vi "Procesado_Matriz.vi"(8 "error in (no error)":errorcluster, 11 "data in":string) -> (0 "error out":errorcluster, 1 "element":u32, 2 "subarray 2":u16[](array[numeric]), 3 "subarray":u16[](array[numeric]))   [LabVIEW 2024]
panel:
  in  "data includes array or string size? (T)":bool=TRUE
  out "*(type *) &x 2":u16[](array[numeric])
  out "*(type *) &x":u8[](array[numeric])
  out "length":i32
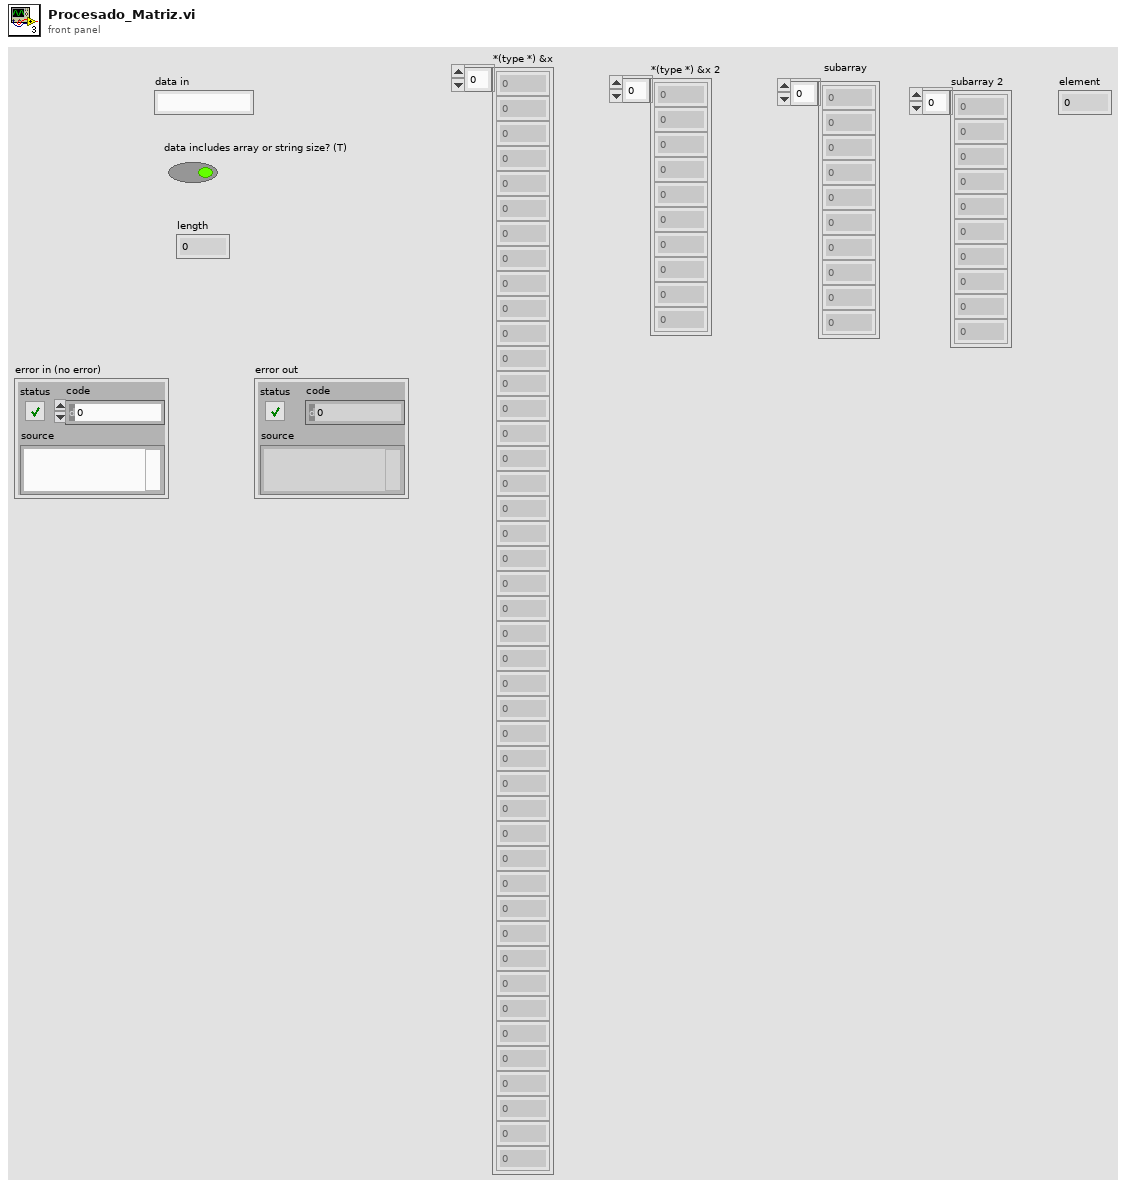
[diagram p1: front panel]
types:
  T1 = enum16{"big-endian, network order", "native, host order", "little-endian"}
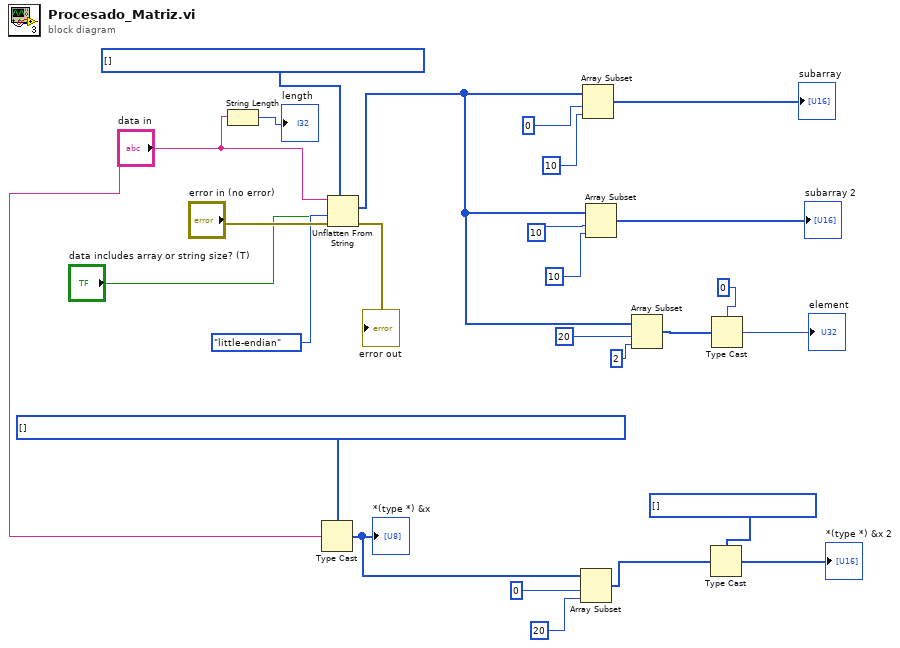
[diagram p0: block diagram]
diagram:
  n1 = String Length(string="data in") -> (length=→"length":i32)
  n2 = Type Cast(type=u8[] [], x="data in") -> (*(type *) &x=w7:u8[])
  "*(type *) &x" <- w7
  n3 = Unflatten From String(type=u16[] [], binary string="data in", data includes array or string size? (T)="data includes array or string size? (T)", byte order (0:big-endian, network order)=T1."little-endian", error in (no error)="error in (no error)") -> (value=w6:u16[], error out=→"error out":errorcluster)  [unwired: 1 out]
  n4 = Array Subset(array=w7, index=0, length=20) -> (w11:u8[])
  n5 = Array Subset(array=w6, index=0, length=10) -> (→"subarray":u16[])
  n6 = Array Subset(array=w6, index=10, length=10) -> (→"subarray 2":u16[])
  n7 = Array Subset(array=w6, index=20, length=2) -> (w2:u16[])
  n8 = Type Cast(type=u16[] [], x=w11) -> (*(type *) &x=→"*(type *) &x 2":u16[])
  n9 = Type Cast(type=u32 0, x=w2) -> (*(type *) &x=→"element":u32)
